vi "Scaner Panel.vi"(8 "error in (no error)":errorcluster, 10 "VISA in":T1={"VISA"="", "baud rate"=9600, "data bits"=8, "parity"=enum."None", "stop bits"=10, "flow control"=0} {"flow control" items=["None", "XON/XOFF", "RTS/CTS", "XON/XOFF & RTS/CTS", "DTR/DSR", "XON/XOFF & DTR/DSR"]; "stop bits" items=["1.0"=10, "1.5"=15, "2.0"=20]}, 11 "Base path":path) -> (0 "error out":errorcluster, 3 "VISA out":T1={"VISA"="", "baud rate"=9600, "data bits"=8, "parity"=enum."None", "stop bits"=10, "flow control"=0} {"flow control" items=["None", "XON/XOFF", "RTS/CTS", "XON/XOFF & RTS/CTS", "DTR/DSR", "XON/XOFF & DTR/DSR"]; "stop bits" items=["1.0"=10, "1.5"=15, "2.0"=20]})   [LabVIEW 2014]
uses:
  SubVI's/VISA/Ctr/VISA Ctr.ctl
panel:
  in  "Cancel":bool
  in  "Save":bool
  in  "VISA":T2={"Visa name"="", "baud rate"=9600, "data bits"=8, "parity"=enum."None", "stop bits"=10, "flow control"=0} {"flow control" items=["None", "XON/XOFF", "RTS/CTS", "XON/XOFF & RTS/CTS", "DTR/DSR", "XON/XOFF & DTR/DSR"]; "stop bits" items=["1.0"=10, "1.5"=15, "2.0"=20]}
  # "Scaner Config"
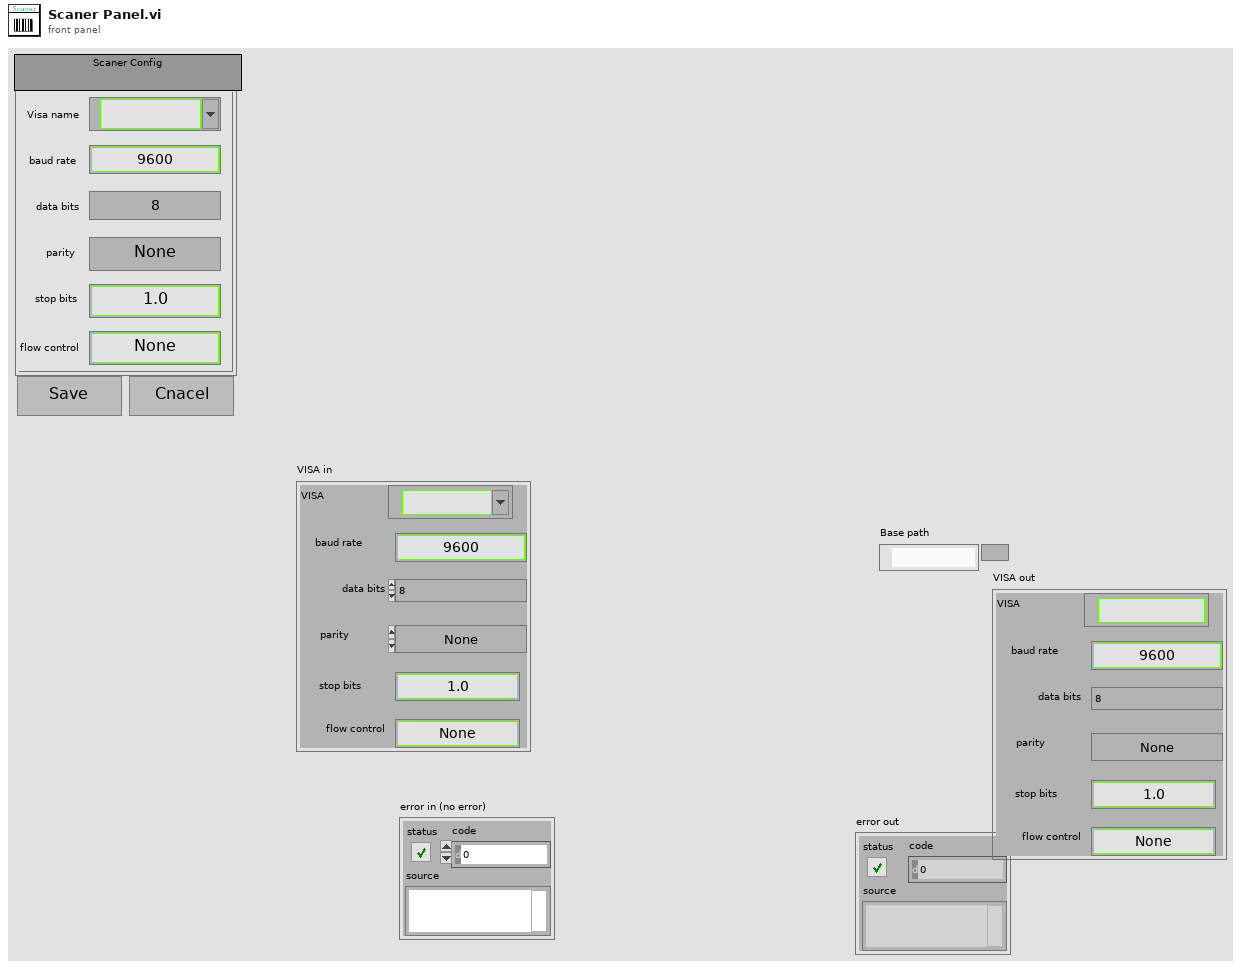
[diagram p1: front panel]
types:
  T1 = typedef "VISA Ctr.ctl" = cluster{"VISA":refnum<visa-resource-name>, "baud rate":u32, "data bits":u16, "parity":enum16{"None", "Odd", "Even", "Mark", "Space"}, "stop bits":u16, "flow control":u16}
  T2 = cluster{"Visa name":refnum<visa-resource-name>, "baud rate":u32, "data bits":u16, "parity":enum16{"None", "Odd", "Even", "Mark", "Space"}, "stop bits":u16, "flow control":u16}
  T3 = cluster{"VISA":refnum<vi>, "VISA in":T1, "Base path":path}
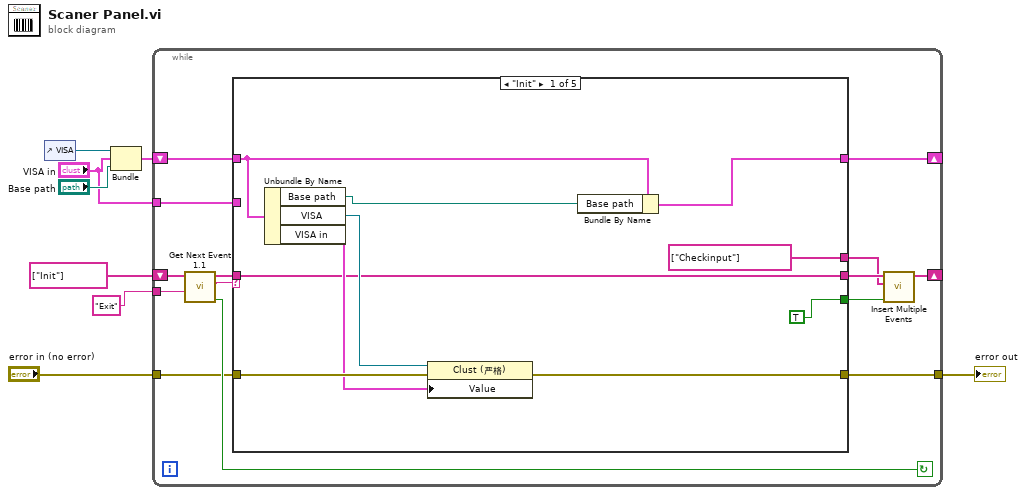
[diagram p0: block diagram]
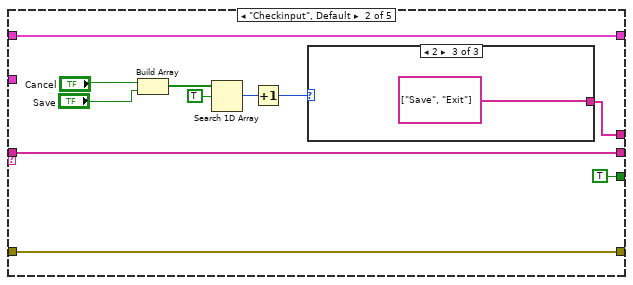
[diagram p2: hidden frame]
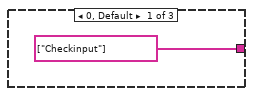
[diagram p3: hidden frame]
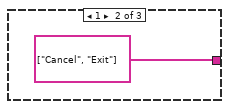
[diagram p4: hidden frame]
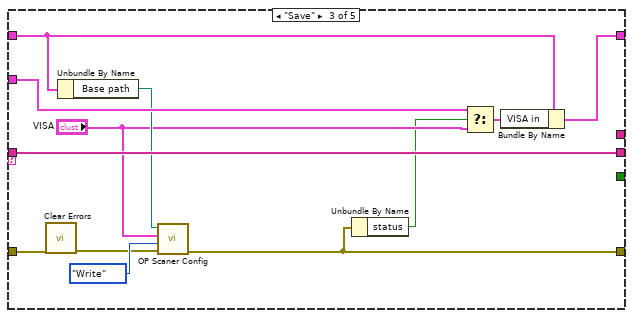
[diagram p5: hidden frame]
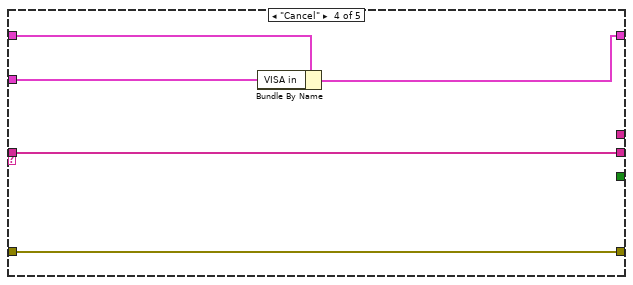
[diagram p6: hidden frame]
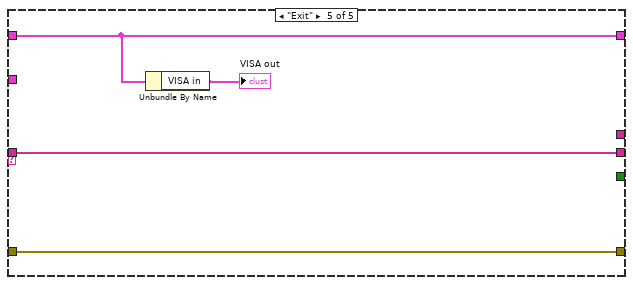
[diagram p7: hidden frame]
diagram:
  n1 = control-ref of="VISA"() -> (w5:refnum<vi>)
  n2 = Bundle("VISA"=w5, "VISA in"="VISA in", "Base path"="Base path") -> (w3:T3)  [unwired: 1 in]
  n3 = while {
    tunnel: "error in (no error)" -> [w16]
    tunnel: "Exit" -> [w21]
    shift-right: [w14] -> _
    shift-left: string[] ["Init"] ("event queue in") -> [w20]
    shift-right: [w10] -> _
    shift-left: w3 -> [w17]
    tunnel: [w15] -> w2
    tunnel: "VISA in" -> [w9]
    stop <- w18 continue-if-true
    n4 = call "Get Next Event 1.1.vi"("Exit Event"=w21, "event queue in"=w20) -> ("Condition (Exit:F)"=w18:bool, "next event"=w22:string, "event queue out"=w19:string[])  [unwired: 6 in, 1 out]
    n5 = case shown="\"Init\"" w22 {
      tunnel: w19 -> [w28 w42 w58 w59 w65]
      tunnel: w17 -> [w25 w43 w55 w62 w67]
      tunnel: w16 -> [w32 w34 w48 w63 w64]
      tunnel: [w29 w34 w50 w63 w64] -> w15
      tunnel: [w28 w42 w58 w59 w65] -> w13
      tunnel: [TRUE TRUE _ _ _] -> w12
      tunnel: [string[] ["Checkinput"] ("event queue in") w35 _ _ _] -> w11
      tunnel: [w24 w43 w54 w60 w67] -> w10
      tunnel: w9 -> [_ _ w57 w61 _]
      frame "Init" {
        n6 = Unbundle By Name(w25) -> ("Base path"=w23:path, "VISA"=w31:refnum<vi>, "VISA in"=w30:T1)
        n7 = property class="Clust (严格)"(reference=w31, error in=w32, "Value"=w30) -> (error out=w29:errorcluster)  [unwired: 1 out]
        n8 = Bundle By Name(cluster=w25, "Base path"=w23) -> (w24:T3)
      }
      frame "Checkinput", Default {
        n9 = Build Array("Cancel", "Save") -> (w39:bool[])
        n10 = Search 1D Array(1D array=w39, element=TRUE) -> (index of element=w37:i32)  [unwired: 1 in]
        n11 = Increment(x=w37) -> (x+1=w36:i32)
        n12 = case shown="2" w36 {
          tunnel: [string[] ["Checkinput"] ("event queue in") string[] ["Cancel", "Exit"] ("event queue in") string[] ["Save", "Exit"] ("event queue in")] -> w35
          frame 0, Default {
          }
          frame 1 {
          }
          frame 2 {
          }
        }
      }
      frame "Save" {
        n13 = call <vilib>:"Clear Errors.vi"("error in (no error)"=w48) -> ("error out"=w47:errorcluster)  [unwired: 5 in, 1 out]
        n14 = Unbundle By Name(w55) -> ("Base path"=w53:path)
        n15 = call "OP Scaner Config.vi"("error in (no error)"=w47, "Enum"=enum16{"init", "Read", "Write"}."Write", "VISA in"="VISA", "Path"=w53) -> ("error out"=w50:errorcluster)  [unwired: 5 in, 2 out]
        n16 = Unbundle By Name(w50) -> ("status"=w49:bool)
        n17 = Select(t=w57, s=w49, f="VISA") -> (s? t:f=w56:T1)
        n18 = Bundle By Name(cluster=w55, "VISA in"=w56) -> (w54:T3)
      }
      frame "Cancel" {
        n19 = Bundle By Name(cluster=w62, "VISA in"=w61) -> (w60:T3)
      }
      frame "Exit" {
        n20 = Unbundle By Name(w67) -> ("VISA in"=→"VISA out":T1)
      }
    }
    n21 = call "Insert Multiple Events.vi"("Insert all? (T)"=w12, "Events to Insert"=w11, "Event queue in"=w13) -> ("Event queue out"=w14:string[])  [unwired: 4 in]
  }
  "error out" <- w2
